vi "posthoc start delay correction.vi"() -> ()   [LabVIEW 2012]
doc: "SciScan 1.2 160622"
uses:
  GFG/GFGnumericGet.vi
  GFG/GFG library.lvlib
panel:
  in  "stop 2":bool
  out "Slide":dbl(slide) caption="SAVING LINESSHIFTED RAW FILE" scale=-1.0..10000.0
  in  "stop":bool
  in  "shift lines by":i32
  out "Image":T1(plugin-control)
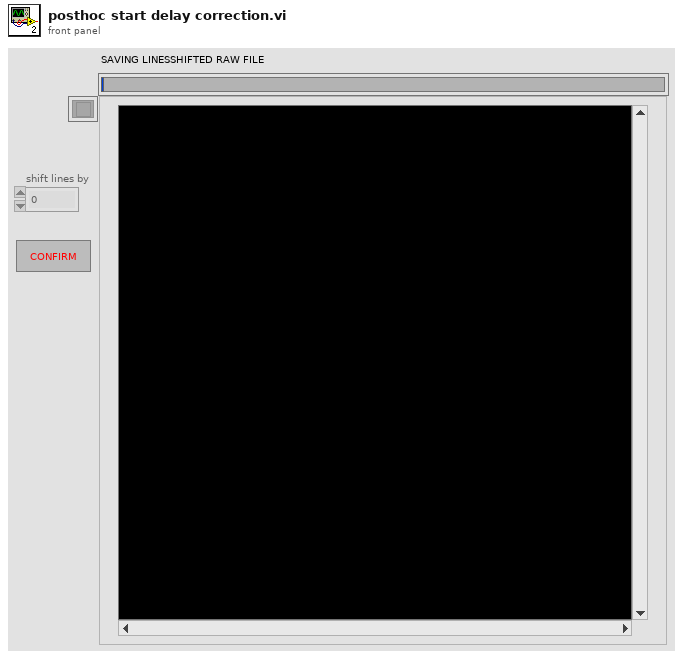
[diagram p1: front panel]
types:
  T1 = typedef "IMAQ Image.ctl" = refnum<image>
  T2 = enum16{"open", "replace", "create", "open or create", "replace or create", "replace or create with confirmation"}
  T3 = enum8{"Enabled", "Disabled", "Disabled and Grayed Out"}
  T4 = typedef "Image Type" = u32
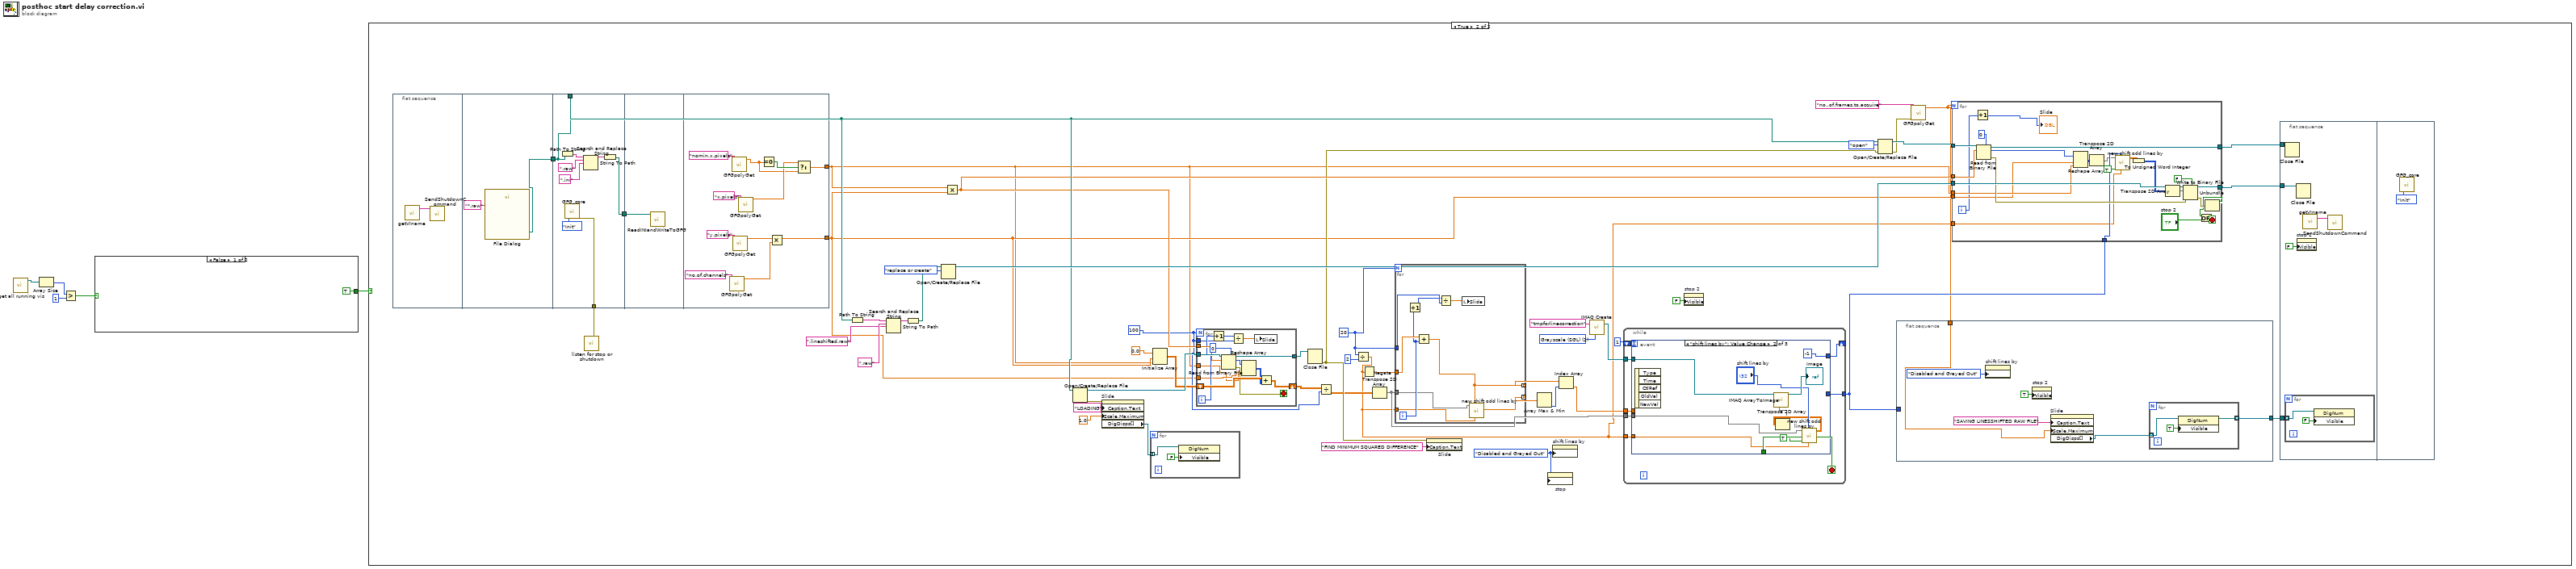
[diagram p0: block diagram]
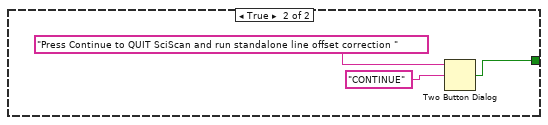
[diagram p2: hidden frame]
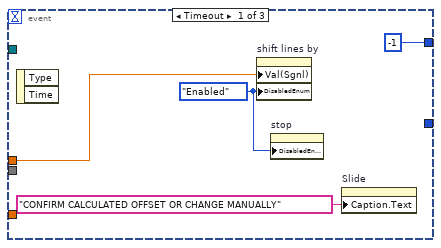
[diagram p4: hidden frame]
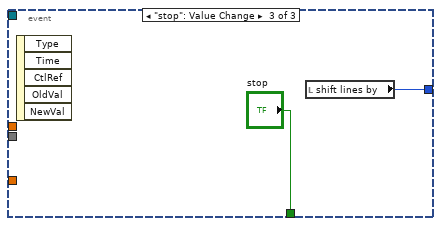
[diagram p5: hidden frame]
diagram:
  n1 = call "get all running vis.vi"() -> ("RunningVIRefs"=w5:refnum<vi>[])  [unwired: 11 in]
  n2 = Array Size(array=w5) -> (size(s)=w4:i32)
  n3 = Greater?(x=w4, y=1) -> (0:w2:bool)
  n4 = case shown="False" w2 {
    tunnel: [TRUE ("T button?") w7] -> w1
    frame False {
    }
    frame True {
      n5 = Two Button Dialog(message="Press Continue to QUIT SciScan and run standalone line offset correction ", 2:"CONTINUE" ("T button name (\"OK\")")) -> (T button?=w7:bool)  [unwired: 1 in]
    }
  }
  n6 = case shown="True" w1 {
    frame False {
    }
    frame True {
      w23 = T3."Disabled and Grayed Out" ("Disabled")
      w29 = 20
      w28 = 100
      w57 = T4 2 items=["Grayscale (U8)", "Grayscale (I16)", "Grayscale (SGL)", "Complex (CSG)", "RGB (U32)", "HSL (U32)", "RGB (U64)", "Grayscale (U16)"] ("Image Type")
      n7 = flat-sequence {
        tunnel: [w153] -> w60
        tunnel: [w161] -> w55
        tunnel: w60 -> [w155]
        tunnel: [w156] -> w59
        tunnel: [w155] -> w47
        tunnel: w59 -> [w163]
        tunnel: [w168] -> w18
        tunnel: [w165] -> w19
        frame #0 {
          n8 = call "getVIname.vi"() -> ("VI name"=w152:string)  [unwired: 19 in]
          n9 = call "SendShutdownCommand.vi"("Source VI"=w152) -> ()  [unwired: 11 in]
        }
        frame #1 {
          n10 = call "File Dialog"("pattern (all files)"="*.raw") -> ("selected path"=w153:path)  [unwired: 11 in, 3 out]
        }
        frame #2 {
          n11 = Path To String(path=w155) -> (string=w160:string)
          n12 = call "GFG_core.vi"("Action"=enum16{"Init", "Set", "Get"}."Init") -> ("error out"=w161:errorcluster)  [unwired: 12 in, 6 out]
          n13 = Search and Replace String(input string=w160, search string=".raw", replace string=".ini" ("replace string (\"\")")) -> (result string=w157:string)  [unwired: 5 in, 3 out]
          n14 = String To Path(string=w157) -> (path=w156:path)
        }
        frame #3 {
          n15 = call "ReadINIandWriteToGFG.vi"("configuration file path"=w163) -> ()  [unwired: 10 in, 1 out]
        }
        frame #4 {
          n16 = call-poly "GFGpolyGet.vi"("Variable Name in"="no.of.channels") -> ("Numeric"=w164:dbl)  [unwired: 8 in, 2 out]
          n17 = call-poly "GFGpolyGet.vi"("Variable Name in"="nomin.x.pixels") -> ("Numeric"=w169:dbl)  [unwired: 8 in, 2 out]
          n18 = call-poly "GFGpolyGet.vi"("Variable Name in"="y.pixels") -> ("Numeric"=w167:dbl)  [unwired: 8 in, 2 out]
          n19 = call-poly "GFGpolyGet.vi"("Variable Name in"="x.pixels") -> ("Numeric"=w170:dbl)  [unwired: 8 in, 2 out]
          n20 = Equal To 0?(x=w169) -> (x = 0?=w171:bool)
          n21 = Multiply(x=w167, y=w164) -> (x*y=w165:dbl)
          n22 = Select(t=w170, s=w171, f=w169) -> (s? t:f=w168:dbl)
        }
      }
      n23 = call "listen for stop or shutdown.vi"("error in (no error)"=w55) -> ()  [unwired: 9 in, 2 out]
      n24 = Path To String(path=w47) -> (string=w52:string)
      n25 = Search and Replace String(input string=w52, search string=".raw", replace string=".lineshifted.raw" ("replace string (\"\")")) -> (result string=w54:string)  [unwired: 5 in, 3 out]
      n26 = String To Path(string=w54) -> (path=w50:path)
      n27 = Open/Create/Replace File(file path (use dialog)=w50, operation (0:open)=T2."replace or create") -> (refnum out=w56:refnum<file>)  [unwired: 4 in, 2 out]
      n28 = Multiply(x=w18, y=w19) -> (x*y=w46:dbl)
      n29 = Open/Create/Replace File(file path (use dialog)=w47) -> (refnum out=w48:refnum<file>, error out=w27:errorcluster)  [unwired: 5 in, 1 out]
      n30 = property on="Slide" class="Slide (strict)"(error in=w27, "Caption.Text"="LOADING", "Scale.Maximum"=1.0 ("Scale.Range:Maximum")) -> ("DigDisps[]"=w12:refnum<vi>[])  [unwired: 1 in, 2 out]
      n31 = for {
        tunnel: w12 -> [w61] mode=indexing
        n32 = property class="DigNum"(reference=w61, "Visible"=FALSE) -> ()  [unwired: 1 in, 2 out]
      }
      n33 = Initialize Array(0.0 ("Numeric"), w19, w18) -> (w44:dbl[][])
      n34 = for {
        N: w28 -> [_]
        tunnel: w48 -> [w151]
        tunnel: w46 -> [w149]
        tunnel: w18 -> [w138]
        tunnel: w19 -> [w139]
        tunnel: [w147] -> w49
        shift-right: [w144] -> w36
        shift-left: w44 -> [w146]
        tunnel: w28 -> [w140]
        i -> [w141]
        stop <- w143 stop-if-true
        n35 = Increment(x=w141) -> (x+1=w137:i32)
        n36 = Read from Binary File(5:u16 0 ("element"), 10:w149, 11:w151) -> (0:w143:errorcluster, 2:w148:u16[], 3:w147:refnum<file>)  [unwired: 3 in, 1 out]
        n37 = Divide(x=w137, y=w140) -> (x/y=w142:dbl)
        n38 = Reshape Array(w148, w139, w138) -> (w145:u16[][])
        n39 = local write "Slide"(w142) -> ()
        n40 = Add(x=w146, y=w145) -> (x+y=w144:dbl[][])
      }
      n41 = Close File(refnum=w49) -> (error out=w24:errorcluster)  [unwired: 1 in, 1 out]
      n42 = Divide(x=w36, y=w28) -> (x/y=w20:dbl[][])
      n43 = Divide(x=w29, y=2) -> (x/y=w14:dbl)
      n44 = Negate(x=w14) -> (-x=w42:dbl)
      n45 = Transpose 2D Array(2D array=w20) -> (transposed array=w17:dbl[][])
      n46 = for {
        N: w29 -> [_]
        tunnel: w42 -> [w136]
        tunnel: w17 -> [w131]
        tunnel: [w129] -> w41 mode=indexing
        tunnel: [w130] -> w40 mode=indexing
        tunnel: w29 -> [w134]
        tunnel: w14 -> [w132]
        i -> [w135]
        n47 = Increment(x=w135) -> (x+1=w128:i32)
        n48 = Add(x=w136, y=w135) -> (x+y=w130:dbl)
        n49 = Divide(x=w128, y=w134) -> (x/y=w133:dbl)
        n50 = local write "Slide"(w133) -> ()
        n51 = call "new shift odd lines by.vi"("max pix shift"=w132, "shift odd lines by"=w130, "pixel array in (x is first dimension)"=w131) -> ("squared difference"=w129:dbl)  [unwired: 7 in, 1 out]
      }
      n52 = property on="Slide" class="Slide (strict)"(error in=w24, "Caption.Text"="FIND MINIMUM SQUARED DIFFERENCE") -> ()  [unwired: 1 in, 2 out]
      n53 = Array Max & Min(array=w41) -> (min index (indices)=w39:i32)  [unwired: 3 out]
      n54 = property on="stop" class="Bool"("DisabledEnum"=w23) -> ()  [unwired: 2 in, 2 out]
      n55 = property on="shift lines by" class="DigNum (strict)"("DisabledEnum"=w23) -> ()  [unwired: 2 in, 2 out]
      n56 = Index Array(array=w40, index=w39) -> (element=w37:dbl)
      n57 = call "IMAQ Create"("Image Name"="tmpforlinecorrection", "Image Type"=w57) -> ("New Image"=w38:T1)  [unwired: 3 in, 1 out]
      n58 = while {
        tunnel: w38 -> [w112]
        tunnel: w17 -> [w110]
        tunnel: w37 -> [w109]
        shift-right: [w107] -> _
        shift-left: 1 -> [w108]
        tunnel: [w106] -> w22
        tunnel: w14 -> [w105]
        stop <- w111 stop-if-true
        n59 = event shown="[1] \"shift lines by\": Value Change" {
          selector: _ -> [_ _ _]
          dyn-events: _ -> [_ _ _]
          timeout: w108 -> [_ _ _]
          tunnel: w112 -> [_ w124 _]
          tunnel: [_ _ "stop"] -> w111
          tunnel: w110 -> [_ w120 _]
          tunnel: w109 -> [w116 _ _]
          tunnel: [-1 -1 _] -> w107
          tunnel: [_ _ w126] -> w106
          tunnel: w105 -> [_ w122 _]
          event Timeout {
            w114 = T3."Enabled" ("Disabled")
            n60 = event-data() -> ()  [unwired: 1 in, 2 out]
            n61 = property on="shift lines by" class="DigNum (strict)"("Val(Sgnl)"=w116, "DisabledEnum"=w114) -> ()  [unwired: 2 in, 2 out]
            n62 = property on="stop" class="Bool"("DisabledEnum"=w114) -> ()  [unwired: 2 in, 2 out]
            n63 = property on="Slide" class="Slide (strict)"("Caption.Text"="CONFIRM CALCULATED OFFSET OR CHANGE MANUALLY") -> ()  [unwired: 2 in, 2 out]
          }
          event "shift lines by": Value Change {
            n64 = event-data() -> ()  [unwired: 1 in, 5 out]
            n65 = call "new shift odd lines by.vi"("max pix shift"=w122, "shift odd lines by"="shift lines by", "calculate shited frame"=TRUE ("calculate squared difference"), "pixel array in (x is first dimension)"=w120) -> ("shifted frame out (x is first dimension)"=w119:dbl[][])  [unwired: 6 in, 1 out]
            n66 = Transpose 2D Array(2D array=w119) -> (transposed array=w118:dbl[][])
            n67 = call "IMAQ ArrayToImage"("Image Pixels (Float)"=w118, "Image"=w124) -> ("Image Out"=→"Image":T1)  [unwired: 8 in, 1 out]
          }
          event "stop": Value Change {
            n68 = event-data() -> ()  [unwired: 1 in, 5 out]
            n69 = local read "shift lines by"() -> (w126:i32)
          }
        }
      }
      n70 = property on="stop 2" class="Bool"("Visible"=FALSE) -> ()  [unwired: 2 in, 2 out]
      n71 = Open/Create/Replace File(file path (use dialog)=w47, error in=w24, operation (0:open)=T2."open") -> (refnum out=w33:refnum<file>, error out=w10:errorcluster)  [unwired: 3 in, 1 out]
      n72 = flat-sequence {
        tunnel: w22 -> [_]
        tunnel: w15 -> [w65]
        tunnel: [w63] -> w13
        frame #0 {
          n73 = property on="shift lines by" class="DigNum (strict)"("DisabledEnum"=T3."Disabled and Grayed Out" ("Disabled")) -> ()  [unwired: 2 in, 2 out]
          n74 = property on="stop 2" class="Bool"("Visible"=TRUE) -> ()  [unwired: 2 in, 2 out]
          n75 = property on="Slide" class="Slide (strict)"("Caption.Text"="SAVING LINESSHIFTED RAW FILE", "Scale.Maximum"=w65) -> ("DigDisps[]"=w64:refnum<vi>[])  [unwired: 2 in, 2 out]
          n76 = for {
            tunnel: w64 -> [w71] mode=indexing
            tunnel: [w69] -> w63 mode=indexing
            n77 = property class="DigNum"(reference=w71, "Visible"=TRUE) -> (reference out=w69:refnum<vi>)  [unwired: 1 in, 1 out]
          }
        }
      }
      n78 = call-poly "GFGpolyGet.vi"("error in (no error)"=w10, "Variable Name in"="no..of.frames.to.acquire") -> ("Numeric"=w15:dbl)  [unwired: 7 in, 2 out]
      n79 = for {
        N: w15 -> [_]
        tunnel: w33 -> [w104]
        tunnel: w46 -> [w102]
        tunnel: w18 -> [w89]
        tunnel: w19 -> [w88]
        tunnel: [w100] -> w32
        tunnel: w56 -> [w97]
        tunnel: [w95] -> w31
        tunnel: w22 -> [w86]
        tunnel: w14 -> [w80]
        i -> [w83]
        stop <- w92 stop-if-true
        n80 = Increment(x=w83) -> (x+1=→"Slide":i32)
        n81 = Read from Binary File(5:u16 0 ("element"), 10:w102, 11:w104) -> (0:w94:errorcluster, 2:w101:u16[], 3:w100:refnum<file>)  [unwired: 3 in, 1 out]
        n82 = Reshape Array(w101, w88, w89) -> (w99:u16[][])
        n83 = Transpose 2D Array(2D array=w99) -> (transposed array=w85:u16[][])
        n84 = call "new shift odd lines by.vi"("max pix shift"=w80, "shift odd lines by"=w86, "calculate shited frame"=TRUE, "pixel array in (x is first dimension)"=w85) -> ("shifted frame out (x is first dimension)"=w84:dbl[][])  [unwired: 6 in, 1 out]
        n85 = To Unsigned Word Integer(number=w84) -> (unsigned 16bit integer=w96:u16[][])
        n86 = Transpose 2D Array(2D array=w96) -> (transposed array=w87:u16[][])
        n87 = Write to Binary File(file (use dialog)=w97, data=w87, error in=w94, 5:FALSE ("prepend array or string size? (T)")) -> (refnum out=w95:refnum<file>, error out=w91:errorcluster)  [unwired: 2 in, 1 out]
        n88 = Unbundle(w91) -> ("status"=w90:bool)  [unwired: 2 out]
        n89 = Or(x=w90, y="stop 2") -> (x .or. y?=w92:bool)
      }
      n90 = flat-sequence {
        tunnel: w32 -> [w76]
        tunnel: w31 -> [w75]
        tunnel: w13 -> [w72]
        frame #0 {
          n91 = Close File(refnum=w76) -> ()  [unwired: 1 in, 2 out]
          n92 = for {
            tunnel: w72 -> [w77] mode=indexing
            n93 = property class="DigNum"(reference=w77, "Visible"=FALSE) -> ()  [unwired: 1 in, 2 out]
          }
          n94 = Close File(refnum=w75) -> ()  [unwired: 1 in, 2 out]
          n95 = property on="stop 2" class="Bool"("Visible"=FALSE) -> ()  [unwired: 2 in, 2 out]
          n96 = call "getVIname.vi"() -> ("VI name"=w74:string)  [unwired: 19 in]
          n97 = call "SendShutdownCommand.vi"("Source VI"=w74) -> ()  [unwired: 11 in]
        }
        frame #1 {
          n98 = call "GFG_core.vi"("Action"=enum16{"Init", "Set", "Get"}."Init") -> ()  [unwired: 12 in, 7 out]
        }
      }
    }
  }
